vi "io_read_OPC.vi"(6 "Block Logging (F)":bool, 8 "error in":errorcluster, 11 "VISA resource name":refnum<visa-resource-name>) -> (0 "error out":errorcluster, 2 "OPC returned":i32 format="%.0x", 3 "VISA resource name out":refnum<visa-resource-name>)   [LabVIEW 2014, in "rszvl_rsidr_core.lvlib"]
uses:
  rszvl_rsidr_core.lvlib
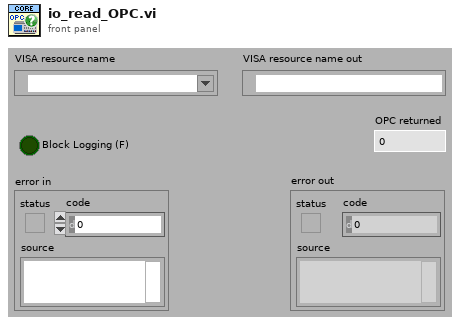
[diagram p1: front panel]
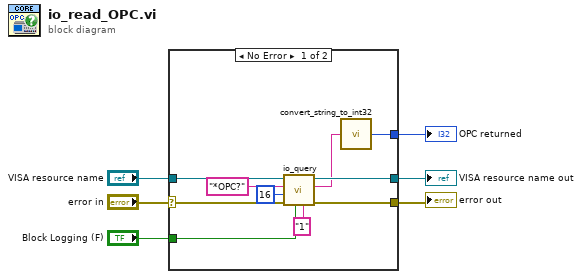
[diagram p0: block diagram]
diagram:
  n1 = case shown="No Error" "error in" {
    selector: "error in" -> [w13 w18]
    tunnel: [w16 w18] -> w6
    tunnel: "VISA resource name" -> [w14 w17]
    tunnel: [w8 _] -> w5
    tunnel: [w15 w17] -> w2
    tunnel: "Block Logging (F)" -> [w7 _]
    frame No Error {
      n2 = call "io_query.vi"("Simulation read buffer (\"Simulation\")"="1" ("Simulation read buffer \n(\"Simulation\")"), "Block Logging (F)"=w7, "error in"=w13, "Bytes to read (2048)"=u32 16 ("Bytes to read (1024)"), "write buffer"="*OPC?", "VISA resource name"=w14) -> ("error out"=w16:errorcluster, "read buffer"=w9:string, "VISA resource name out"=w15:refnum<visa-resource-name>)  [unwired: 2 in, 1 out]
      n3 = call "convert_string_to_int32.vi"("String in"=w9) -> ("int32 value out"=w8:i32)  [unwired: 4 in]
    }
    frame Error {
    }
  }
  "VISA resource name out" <- w2
  "error out" <- w6
  "OPC returned" <- w5
